vi "求取特征系数.vi"(4 "speech":dbl[](array[numeric])) -> (0 "波形图":dbl[](graph), 1 "cof":dbl[][](array[numeric]))   [LabVIEW 2018]
panel:
  out "error out":errorcluster
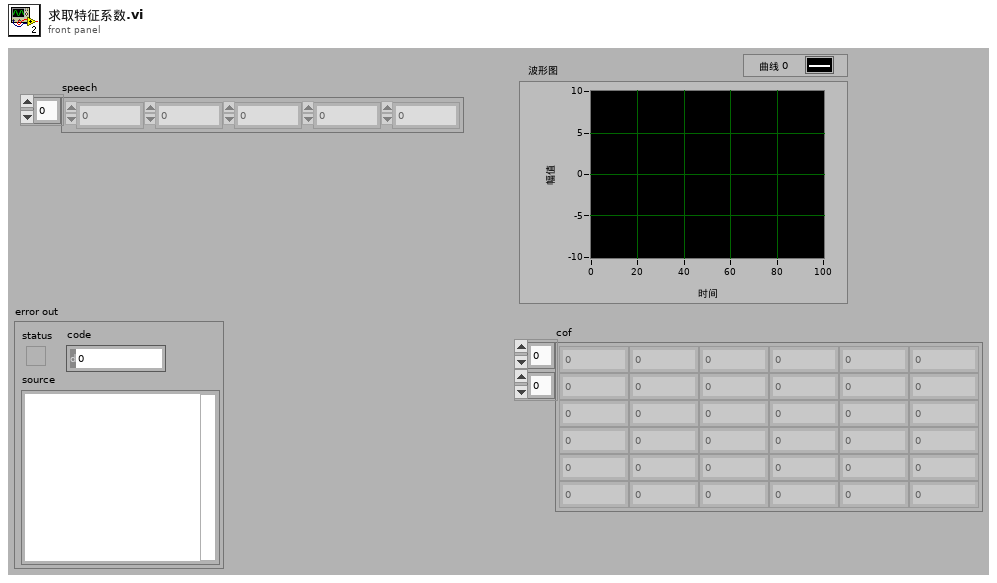
[diagram p1: front panel]
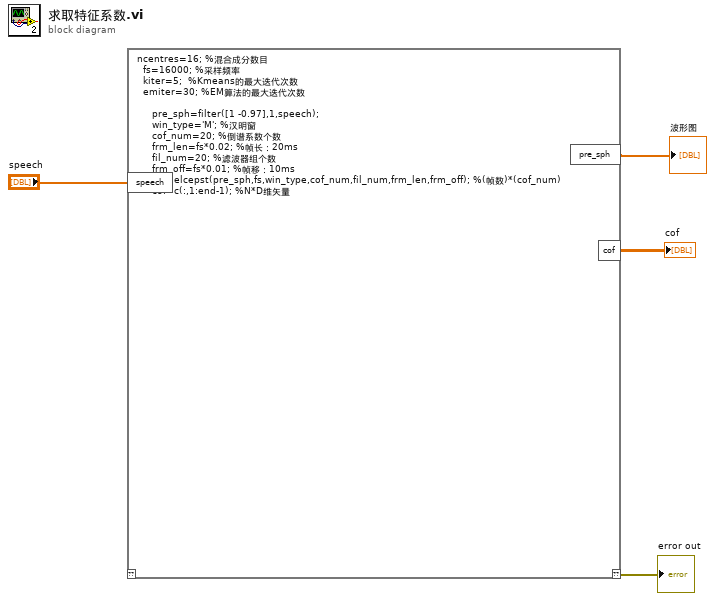
[diagram p0: block diagram]
diagram:
  n1 = script code="ncentres=16; %混合成分数目\n  fs=16000; %采样频率  \n  kiter=5;  %Kmeans的最大迭代次数\n  emiter=30; %EM算法的最大迭代次数\n\n     pre_sph=filter([1 -0.97],1,speech);\n     win_type='M'; %汉明窗\n     cof_num=20; %倒谱系数个数\n     frm_len=fs*0.02; %帧长：20ms\n     fil_num=20; %滤波器组个数\n     frm_off=fs*0.01; %帧移：10ms\n     c=melcepst(pre_sph,fs,win_type,cof_num,fil_num,frm_len,frm_off); %(帧数)*(cof_num)\n     cof=c(:,1:end-1); %N*D维矢量"("speech"="speech") -> ("??"=→"error out":errorcluster, "cof"=→"cof":dbl[][], "pre_sph"=→"波形图":dbl[])  [unwired: 1 in]
